vi "RandomColor.vi"() -> (2 "String":string)   [LabVIEW 2016]
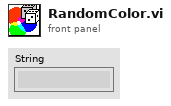
[diagram p1: front panel]
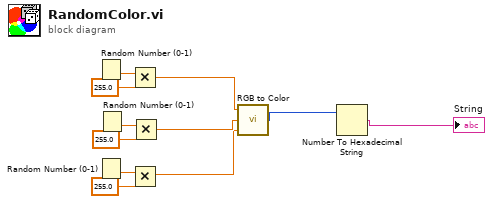
[diagram p0: block diagram]
diagram:
  n1 = Random Number (0-1)() -> (number: 0 to 1=w11:dbl)
  n2 = Random Number (0-1)() -> (number: 0 to 1=w5:dbl)
  n3 = Random Number (0-1)() -> (number: 0 to 1=w8:dbl)
  n4 = Multiply(x=w11, y=255.0) -> (x*y=w9:dbl)
  n5 = Multiply(x=w5, y=255.0) -> (x*y=w3:dbl)
  n6 = Multiply(x=w8, y=255.0) -> (x*y=w4:dbl)
  n7 = call <vilib>:"RGB to Color.vi"("B"=w3, "G"=w4, "R"=w9) -> ("Color"=w2:u32)
  n8 = Number To Hexadecimal String(2:w2) -> (0:→"String":string)  [unwired: 1 in]
